vi "Read.vi"(8 "error in (no error)":errorcluster, 11 "Mock Instrument Interface in":refnum<class "Mock Instrument.lvclass">) -> (0 "error out":errorcluster, 2 "Data":string, 3 "Mock Instrument Interface out":refnum<class "Mock Instrument.lvclass">)   [LabVIEW 2020, in "Low Level PSU With Tests.lvlib" / "Mock Instrument.lvclass"]
uses:
  Mock Instrument.lvclass
  Mock Instrument.lvclass/Mock Instrument.ctl
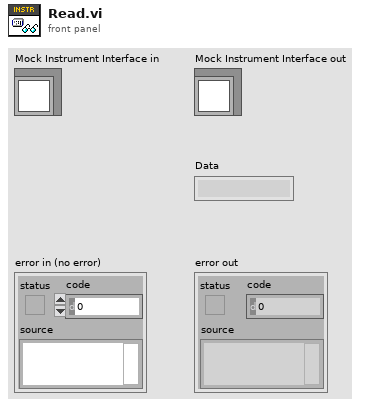
[diagram p1: front panel]
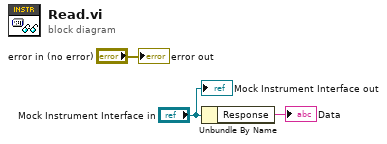
[diagram p0: block diagram]
diagram:
  n1 = Unbundle By Name("Mock Instrument Interface in") -> ("Response"=→"Data":string)
  "error out" <- "error in (no error)"
  "Mock Instrument Interface out" <- "Mock Instrument Interface in"
